vi "lvDiff.vi"   [LabVIEW 2014, in "lv-cli-steps.lvlib"]
uses:
  lv-cli-steps.lvlib
  <vilib>/Utility/error.llb/DialogType.ctl
  <vilib>/lvrevbrd/DiffVIs.lvlib
  <vilib>/Wiresmith Technology/LabVIEW CLI/CLI Class/CLI.lvclass
  <vilib>/lvrevbrd/ScreenshotVI.lvlib
types:
  T1 = typedef "DialogType.ctl" = u16
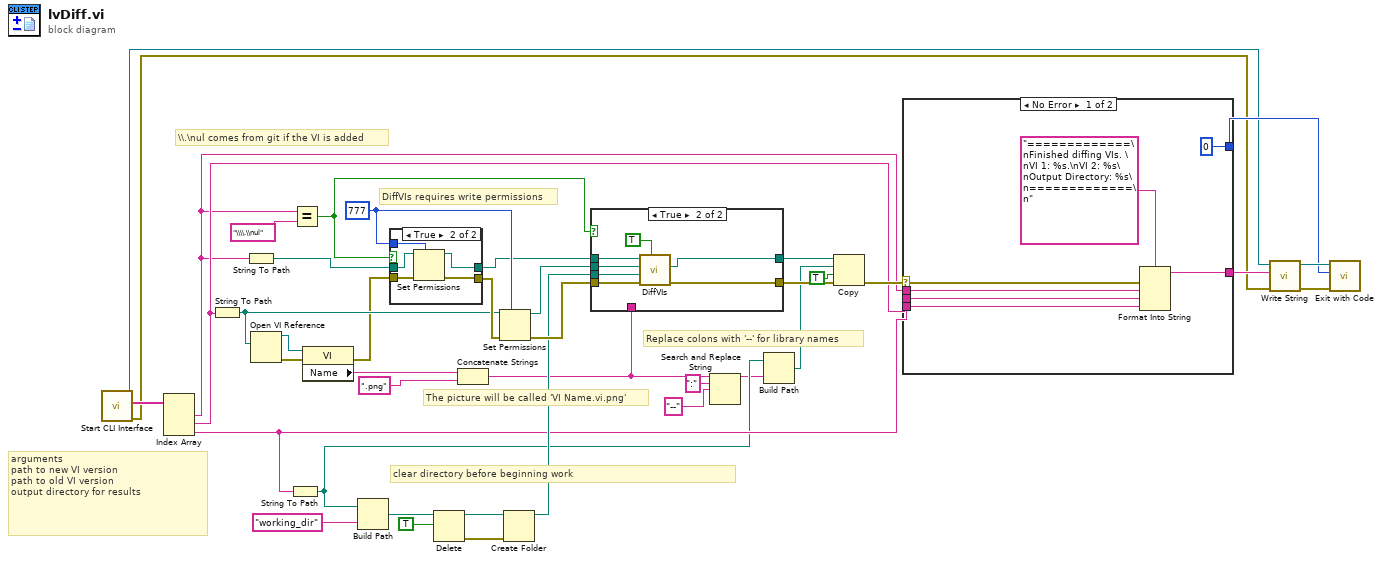
[diagram p0: block diagram]
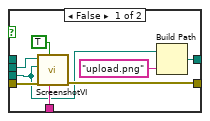
[diagram p3: hidden frame]
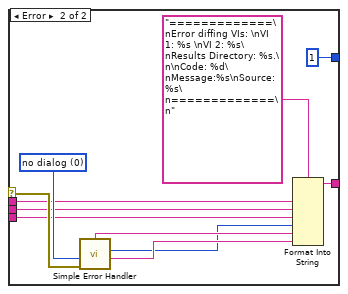
[diagram p4: hidden frame]
diagram:
  w21 = i16 777 ("permissions")
  # "\\\\.\\nul comes from git if the VI is added"
  # "Replace colons with '--' for library names"
  # "clear directory before beginning work"
  # "DiffVIs requires write permissions"
  # "The picture will be called 'VI Name.vi.png'"
  # "arguments\npath to new VI version\npath to old VI version\noutput directory for results"
  n1 = call <vilib>:"Start CLI Interface.vi"() -> ("error out"=w19:errorcluster, "Custom Parameters"=w26:string[], "CLI out"=w27:refnum<class "CLI.lvclass">)  [unwired: 9 in]
  n2 = Index Array(array=w26) -> (element #1=w4:string, element #2=w22:string, element #3=w23:string)  [unwired: 3 in]
  n3 = String To Path(string=w22) -> (path=w17:path)
  n4 = String To Path(string=w4) -> (path=w35:path)
  n5 = Open VI Reference(vi path=w17) -> (vi reference=w16:refnum<vi>, error out=w15:errorcluster)  [unwired: 5 in]
  n6 = String To Path(string=w23) -> (path=w18:path)
  n7 = Equal?(x=w4, y="\\\\.\\nul") -> (x = y?=w2:bool)
  n8 = property class="VI"(reference=w16, error in=w15) -> (error out=w14:errorcluster, "Name"=w13:string)  [unwired: 1 out]
  n9 = Build Path(base path=w18, name or relative path="working_dir") -> (appended path=w11:path)
  n10 = case shown="True" w2 {
    tunnel: w35 -> [w41 w47]
    tunnel: [w42 w46] -> w25
    tunnel: w21 -> [_ w45]
    tunnel: w14 -> [w42 w44]
    tunnel: [w41 w43] -> w1
    frame False {
    }
    frame True {
      n11 = Set Permissions(7:w45, 8:w44, 11:w47) -> (0:w46:errorcluster, 3:w43:path)  [unwired: 2 in]
    }
  }
  n12 = Delete(path (use dialog)=w11, entire hierarchy (F)=TRUE) -> (deleted path=w10:path, error out=w12:errorcluster)  [unwired: 3 in, 1 out]
  n13 = Concatenate Strings(w13, ".png" ("string")) -> (w3:string)
  n14 = Set Permissions(7:w21, 8:w25, 11:w17) -> (0:w40:errorcluster, 3:w39:path)  [unwired: 2 in]
  n15 = Create Folder(path (use dialog)=w10, error in=w12) -> (created path=w37:path)  [unwired: 1 in, 2 out]
  n16 = case shown="True" w2 {
    tunnel: w40 -> [w52 w61]
    tunnel: w39 -> [w53 w60]
    tunnel: [w50 w59] -> w38
    tunnel: w37 -> [w48 w58]
    tunnel: [w54 w57] -> w36
    tunnel: w3 -> [w51 _]
    tunnel: w1 -> [_ w56]
    frame False {
      n17 = call <vilib>:"ScreenshotVI.vi"("Title Prefix In"=w51, "Take Scrshots All In"=TRUE, "error in"=w52, "Picture Save Location"=w48, "VI Path"=w53) -> ("error out"=w54:errorcluster)  [unwired: 3 in, 3 out]
      n18 = Build Path(base path=w48, name or relative path="upload.png") -> (appended path=w50:path)
    }
    frame True {
      n19 = call <vilib>:"DiffVIs.vi"("Take ScrShots All In"=TRUE, "error in"=w61, "Picture Save Location"=w58, "VI Path 2"=w60, "VI Path 1"=w56) -> ("error out"=w57:errorcluster, "diff file"=w59:path)  [unwired: 2 in, 3 out]
    }
  }
  n20 = Search and Replace String(input string=w3, search string=":", replace string="--" ("replace string (\"\")")) -> (result string=w8:string)  [unwired: 5 in, 3 out]
  n21 = Build Path(base path=w18, name or relative path=w8) -> (appended path=w32:path)
  n22 = Copy(8:w36, 9:TRUE ("overwrite (F)"), 10:w32, 11:w38) -> (0:w24:errorcluster)  [unwired: 1 in, 2 out]
  n23 = case shown="No Error" w24 {
    selector: w24 -> [w68 w79]
    tunnel: [w67 w80] -> w31
    tunnel: [0 ("Exit Code (0)") 1 ("Exit Code (0)")] -> w29
    tunnel: w22 -> [w64 w71]
    tunnel: w23 -> [w63 w72]
    tunnel: w4 -> [w65 w70]
    frame No Error {
      n24 = Format Into String(format string="=============\nFinished diffing VIs. \nVI 1: %s.\nVI 2: %s\nOutput Directory: %s\n=============\n", error in=w68, w65, w64, w63) -> (resulting string=w67:string)  [unwired: 1 in, 1 out]
    }
    frame Error {
      w78 = T1 0 items=["no dialog", "OK message", "continue or stop message", "OK message + warnings", "continue/stop + warnings"] ("type of dialog (OK msg:1)")
      n25 = call <vilib>:"Simple Error Handler.vi"("type of dialog (OK msg:1)"=w78, "error in (no error)"=w79) -> ("code out"=w73:i32, "source out"=w74:string, "message"=w75:string)  [unwired: 3 in, 2 out]
      n26 = Format Into String(format string="=============\nError diffing VIs: \nVI 1: %s \nVI 2: %s\nResults Directory: %s.\n\nCode: %d\nMessage:%s\nSource: %s\n=============\n", w70, w71, w72, w73, w75, w74) -> (resulting string=w80:string)  [unwired: 2 in, 1 out]
    }
  }
  n27 = call <vilib>:"Write String.vi"("error in (no error)"=w19, "Text to Write"=w31, "CLI in"=w27) -> ("error out"=w28:errorcluster, "CLI out"=w30:refnum<class "CLI.lvclass">)  [unwired: 7 in]
  n28 = call <vilib>:"Exit with Code.vi"("error in (no error)"=w28, "Exit Code (0)"=w29, "CLI in"=w30) -> ()  [unwired: 8 in, 1 out]
